vi "Initialize Small Field (N.O.).vi"(8 "error in (no error)":errorcluster, 10 "input cluster":T1, 11 "VISA session":refnum<visa-resource-name>) -> (0 "error out":errorcluster, 1 "Positive?":bool, 2 "output cluster":T1, 3 "dup VISA session":refnum<visa-resource-name>)   [LabVIEW 2012]
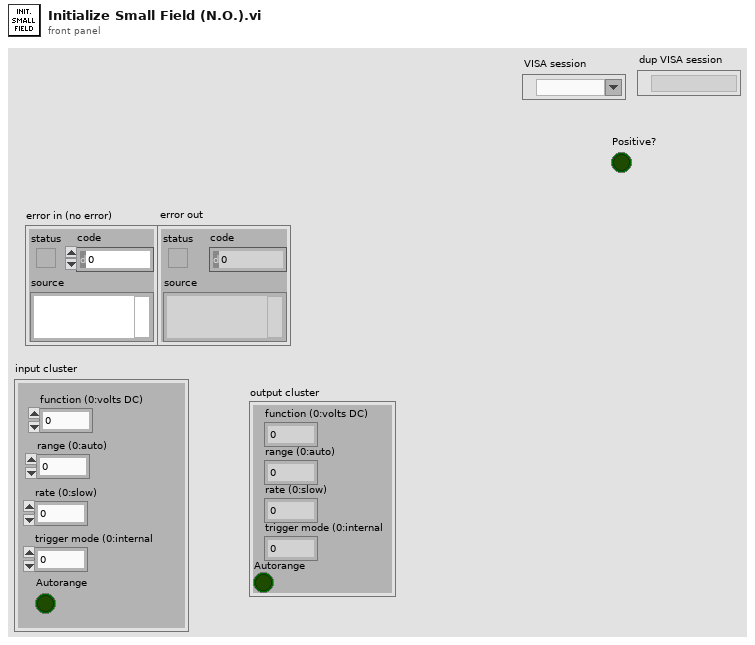
[diagram p1: front panel]
types:
  T1 = cluster{"function (0:volts DC)":i16, "range (0:auto)":i16, "rate (0:slow)":i16, "trigger mode (0:internal":i16, "Autorange":bool}
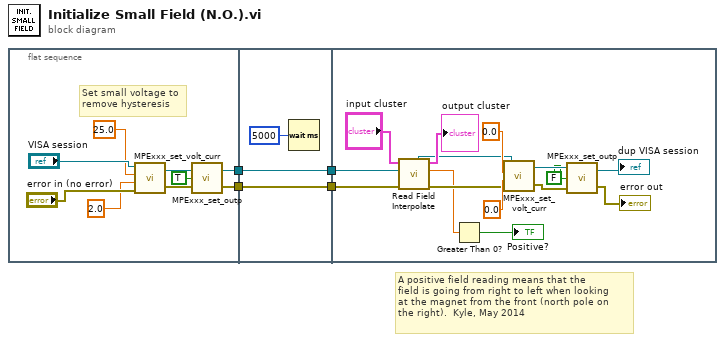
[diagram p0: block diagram]
diagram:
  # "A positive field reading means that the\nfield is going from right to left when looking\nat the magnet from the front (north pole on\nthe right).  Kyle, May 2014"
  n1 = flat-sequence {
    tunnel: [w6] -> w4
    tunnel: [w5] -> w3
    tunnel: w4 -> [w16]
    tunnel: w3 -> [w15]
    tunnel: [w16] -> w2
    tunnel: [w15] -> w1
    tunnel: w2 -> [w18]
    tunnel: w1 -> [w31]
    frame #0 {
      # "Set small voltage to\nremove hysteresis"
      n2 = call "MPExxx_set_volt_curr.vi"("error in (no error)"="error in (no error)", "Set Current"=2.0, "Set Voltage"=25.0, "VISA session"="VISA session") -> ("error out"=w7:errorcluster, "dup VISA session"=w8:refnum<visa-resource-name>)
      n3 = call "MPExxx_set_outp.vi"("error in (no error)"=w7, "Output Control"=TRUE, "VISA session"=w8) -> ("error out"=w5:errorcluster, "dup VISA session"=w6:refnum<visa-resource-name>)
    }
    frame #1 {
      n4 = Wait (ms)(milliseconds to wait=u32 5000) -> ()  [unwired: 1 out]
    }
    frame #2 {
      n5 = call "Read Field Interpolate.vi"("error in (no error)"=w31, "VISA session"=w18, "input cluster"="input cluster") -> ("error out"=w26:errorcluster, "Field (T)"=w19:dbl, "output cluster"=→"output cluster":T1, "dup VISA session"=w17:refnum<visa-resource-name>)  [unwired: 3 in, 2 out]
      n6 = Greater Than 0?(x=w19) -> (x > 0?=→"Positive?":bool)
      n7 = call "MPExxx_set_volt_curr.vi"("error in (no error)"=w26, "Set Current"=0.0, "Set Voltage"=0.0, "VISA session"=w17) -> ("error out"=w22:errorcluster, "dup VISA session"=w23:refnum<visa-resource-name>)
      n8 = call "MPExxx_set_outp.vi"("error in (no error)"=w22, "Output Control"=FALSE, "VISA session"=w23) -> ("error out"=→"error out":errorcluster, "dup VISA session"=→"dup VISA session":refnum<visa-resource-name>)
    }
  }
